vi "Find Block Statistics x8 (SubVI).vi"(0 "Pixel Data":u64, 5 "Pixel Valid?":bool, 8 "Block Size x2":u16=8) -> (14 "Maximum":u8, 16 "Minimum":u8, 19 "Result Valid?":bool)   [LabVIEW 2015]
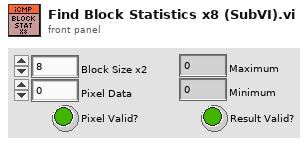
[diagram p1: front panel]
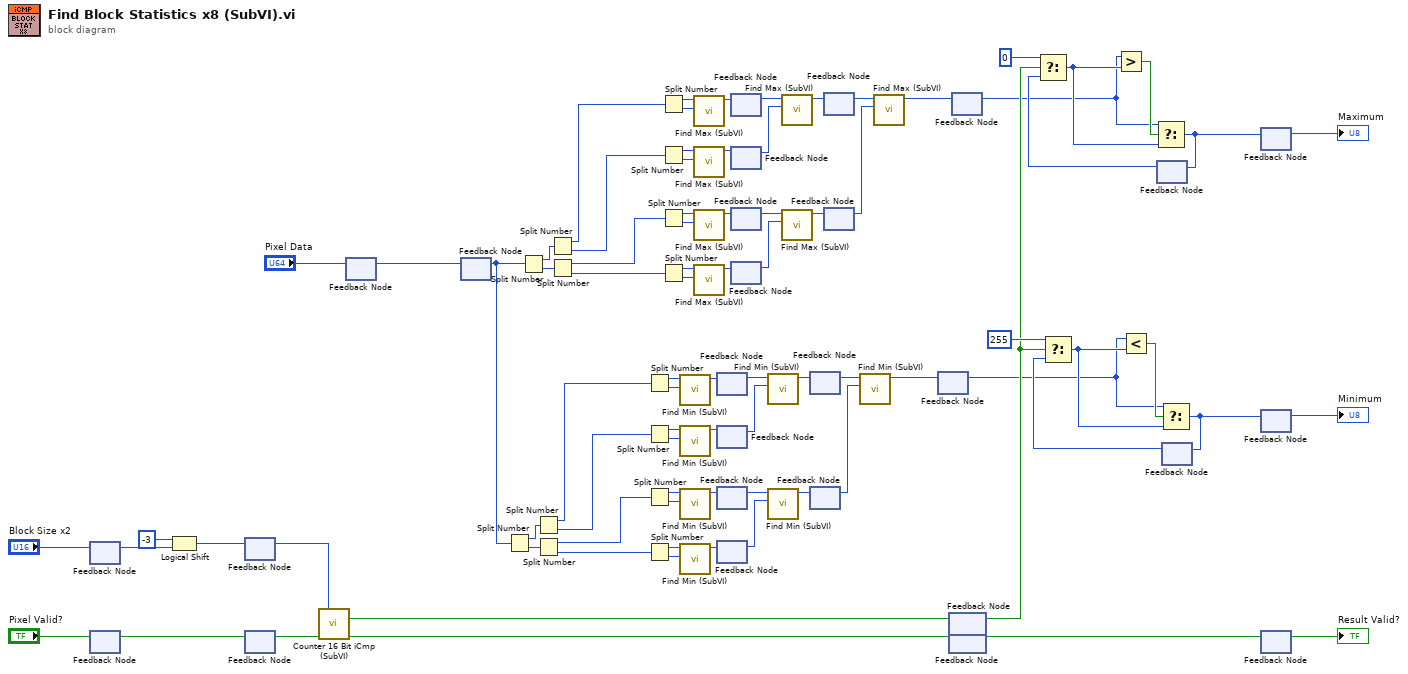
[diagram p0: block diagram]
diagram:
  n1 = feedback-in #1("Block Size x2") -> ()
  n2 = feedback #1() -> (w34:u16)  [unwired: 1 in]
  n3 = feedback-in #2("Pixel Valid?") -> ()
  n4 = feedback #2() -> (w33:bool)  [unwired: 1 in]
  n5 = Logical Shift(y=i16 -3, x=w34) -> (x << y=w69:u16)
  n6 = feedback-in #3(w69) -> ()
  n7 = feedback #3() -> (w67:u16)  [unwired: 1 in]
  n8 = feedback-in #4(w33) -> ()
  n9 = feedback #4() -> (w66:bool)  [unwired: 1 in]
  n10 = call "Counter 16 Bit iCmp (SubVI).vi"("Max. Count"=w67, "Enable"=w66) -> ("Count Begin?"=w81:bool, "Count End?"=w84:bool)  [unwired: 11 in, 1 out]
  n11 = feedback-in #5("Pixel Data") -> ()
  n12 = feedback #5() -> (w35:u64)  [unwired: 1 in]
  n13 = feedback-in #6(w35) -> ()
  n14 = feedback #6() -> (w2:u64)  [unwired: 1 in]
  n15 = Split Number(x=w2) -> (hi(x)=w4:u32, lo(x)=w3:u32)
  n16 = Split Number(x=w2) -> (hi(x)=w64:u32, lo(x)=w65:u32)
  n17 = Split Number(x=w4) -> (hi(x)=w5:u16, lo(x)=w10:u16)
  n18 = Split Number(x=w3) -> (hi(x)=w13:u16, lo(x)=w16:u16)
  n19 = Split Number(x=w64) -> (hi(x)=w63:u16, lo(x)=w58:u16)
  n20 = Split Number(x=w65) -> (hi(x)=w55:u16, lo(x)=w52:u16)
  n21 = Split Number(x=w5) -> (hi(x)=w6:u8, lo(x)=w7:u8)
  n22 = Split Number(x=w10) -> (hi(x)=w9:u8, lo(x)=w8:u8)
  n23 = Split Number(x=w13) -> (hi(x)=w11:u8, lo(x)=w12:u8)
  n24 = Split Number(x=w16) -> (hi(x)=w15:u8, lo(x)=w14:u8)
  n25 = Split Number(x=w63) -> (hi(x)=w62:u8, lo(x)=w61:u8)
  n26 = Split Number(x=w58) -> (hi(x)=w59:u8, lo(x)=w60:u8)
  n27 = Split Number(x=w55) -> (hi(x)=w57:u8, lo(x)=w56:u8)
  n28 = Split Number(x=w52) -> (hi(x)=w53:u8, lo(x)=w54:u8)
  n29 = call "Find Min (SubVI).vi"("Data 2"=w7, "Data 1"=w6) -> ("Min"=w17:u8)  [unwired: 9 in]
  n30 = call "Find Min (SubVI).vi"("Data 2"=w8, "Data 1"=w9) -> ("Min"=w18:u8)  [unwired: 9 in]
  n31 = call "Find Min (SubVI).vi"("Data 2"=w12, "Data 1"=w11) -> ("Min"=w19:u8)  [unwired: 9 in]
  n32 = call "Find Min (SubVI).vi"("Data 2"=w14, "Data 1"=w15) -> ("Min"=w20:u8)  [unwired: 9 in]
  n33 = call "Find Max (SubVI).vi"("Data 2"=w61, "Data 1"=w62) -> ("Max"=w51:u8)  [unwired: 9 in]
  n34 = call "Find Max (SubVI).vi"("Data 2"=w60, "Data 1"=w59) -> ("Max"=w50:u8)  [unwired: 9 in]
  n35 = call "Find Max (SubVI).vi"("Data 2"=w56, "Data 1"=w57) -> ("Max"=w49:u8)  [unwired: 9 in]
  n36 = call "Find Max (SubVI).vi"("Data 2"=w54, "Data 1"=w53) -> ("Max"=w48:u8)  [unwired: 9 in]
  n37 = feedback #7() -> (w23:u8)  [unwired: 1 in]
  n38 = feedback-in #7(w17) -> ()
  n39 = feedback #8() -> (w24:u8)  [unwired: 1 in]
  n40 = feedback-in #8(w18) -> ()
  n41 = feedback #9() -> (w25:u8)  [unwired: 1 in]
  n42 = feedback-in #9(w19) -> ()
  n43 = feedback #10() -> (w26:u8)  [unwired: 1 in]
  n44 = feedback-in #10(w20) -> ()
  n45 = feedback-in #11(w51) -> ()
  n46 = feedback #11() -> (w45:u8)  [unwired: 1 in]
  n47 = feedback-in #12(w50) -> ()
  n48 = feedback #12() -> (w44:u8)  [unwired: 1 in]
  n49 = feedback-in #13(w49) -> ()
  n50 = feedback #13() -> (w43:u8)  [unwired: 1 in]
  n51 = feedback-in #14(w48) -> ()
  n52 = feedback #14() -> (w42:u8)  [unwired: 1 in]
  n53 = call "Find Min (SubVI).vi"("Data 2"=w24, "Data 1"=w23) -> ("Min"=w21:u8)  [unwired: 9 in]
  n54 = call "Find Min (SubVI).vi"("Data 2"=w26, "Data 1"=w25) -> ("Min"=w22:u8)  [unwired: 9 in]
  n55 = call "Find Max (SubVI).vi"("Data 2"=w44, "Data 1"=w45) -> ("Max"=w47:u8)  [unwired: 9 in]
  n56 = call "Find Max (SubVI).vi"("Data 2"=w42, "Data 1"=w43) -> ("Max"=w46:u8)  [unwired: 9 in]
  n57 = feedback #15() -> (w28:u8)  [unwired: 1 in]
  n58 = feedback-in #15(w21) -> ()
  n59 = feedback #16() -> (w27:u8)  [unwired: 1 in]
  n60 = feedback-in #16(w22) -> ()
  n61 = feedback-in #17(w47) -> ()
  n62 = feedback #17() -> (w40:u8)  [unwired: 1 in]
  n63 = feedback-in #18(w46) -> ()
  n64 = feedback #18() -> (w41:u8)  [unwired: 1 in]
  n65 = call "Find Min (SubVI).vi"("Data 2"=w27, "Data 1"=w28) -> ("Min"=w29:u8)  [unwired: 9 in]
  n66 = call "Find Max (SubVI).vi"("Data 2"=w41, "Data 1"=w40) -> ("Max"=w37:u8)  [unwired: 9 in]
  n67 = feedback #19() -> (w1:u8)  [unwired: 1 in]
  n68 = feedback-in #19(w29) -> ()
  n69 = feedback-in #20(w81) -> ()
  n70 = feedback #20() -> (w39:bool)  [unwired: 1 in]
  n71 = feedback-in #21(w84) -> ()
  n72 = feedback #21() -> (w38:bool)  [unwired: 1 in]
  n73 = feedback-in #22(w37) -> ()
  n74 = feedback #22() -> (w36:u8)  [unwired: 1 in]
  n75 = feedback #23() -> (w76:u8)  [unwired: 1 in]
  n76 = Select(t=u8 0, s=w39, f=w76) -> (s? t:f=w71:u8)
  n77 = Greater?(x=w36, y=w71) -> (0:w74:bool)
  n78 = Select(t=w36, s=w74, f=w71) -> (s? t:f=w83:u8)
  n79 = feedback-in #23(w83) -> ()
  n80 = feedback #24() -> (w77:u8)  [unwired: 1 in]
  n81 = Select(t=u8 255, s=w39, f=w77) -> (s? t:f=w70:u8)
  n82 = Less?(x=w1, y=w70) -> (x < y?=w79:bool)
  n83 = Select(t=w1, s=w79, f=w70) -> (s? t:f=w82:u8)
  n84 = feedback-in #24(w82) -> ()
  n85 = feedback-in #25(w83) -> ()
  n86 = feedback #25() -> (→"Maximum":u8)  [unwired: 1 in]
  n87 = feedback-in #26(w82) -> ()
  n88 = feedback #26() -> (→"Minimum":u8)  [unwired: 1 in]
  n89 = feedback-in #27(w38) -> ()
  n90 = feedback #27() -> (→"Result Valid?":bool)  [unwired: 1 in]
